vi "RT Loop - Watchdog.vi"(10 "FPGA VI Reference(Old)":T1, 11 "Message Queue":refnum<queue>) -> ()   [LabVIEW 2013]
uses:
  support/Message Queue/Message Cluster.ctl
  controls/FPGA VI Reference.ctl
  Globals/Global - Configuration Options.vi
  <vilib>/Utility/error.llb/Error Cluster From Error Code.vi
  <vilib>/rvi/errors/niLvFpgaAdjustHostInterfaceError.vi
  Globals/Global - All RT Loop Stop.vi
  <vilib>/rvi/interface/nirviReadWriteControl/nirviReadWriteControl.xnode
  FPGA Bitfiles/crio-FPGA-contro_FPGATarget_FPGAMain_4HKUk4gb9wY.lvbitx
  NiFpgaLv.dll
  support/Message Queue/Message Queue.lvlib
panel:
  in  "FPGA VI Reference":refnum<k20>
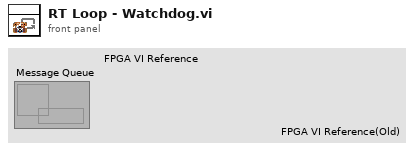
[diagram p1: front panel]
types:
  T1 = typedef "FPGA VI Reference.ctl" = refnum<k20>
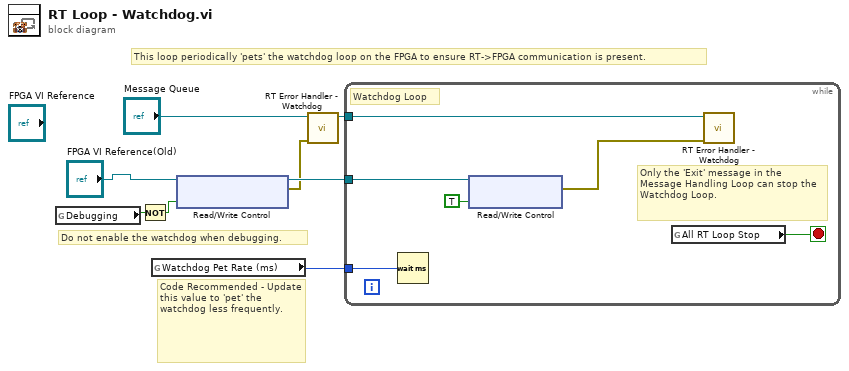
[diagram p0: block diagram]
diagram:
  # "Do not enable the watchdog when debugging."
  # "Code Recommended - Update this value to 'pet' the watchdog less frequently."
  # "This loop periodically 'pets' the watchdog loop on the FPGA to ensure RT->FPGA communication is present."
  n1 = global read "Global - Configuration Options.vi" "Debugging"() -> (w3:bool)
  n2 = Not(x=w3) -> (.not. x?=w2:bool)
  n3 = global read "Global - Configuration Options.vi" "Watchdog Pet Rate (ms)"() -> (w8:u32)
  n4 = xnode "Read/Write Control"("FPGA VI Reference In"="FPGA VI Reference(Old)", "Enable Watchdog"=w2) -> ("FPGA VI Reference Out"=w7:T1, "error out"=w4:errorcluster)  [unwired: 1 in]
  n5 = call "RT Error Handler - Watchdog.vi"("error in (no error)"=w4, "Message Queue"="Message Queue") -> ("dup Message Queue"=w5:refnum<queue>)  [unwired: 9 in]
  n6 = while {
    tunnel: w5 -> [w11]
    tunnel: w7 -> [w14]
    tunnel: w8 -> [w9]
    stop <- w12 stop-if-true
    # "Only the 'Exit' message in the  Message Handling Loop can stop the Watchdog Loop."
    # "Watchdog Loop"
    n7 = Wait (ms)(milliseconds to wait=w9) -> ()  [unwired: 1 out]
    n8 = xnode "Read/Write Control"("FPGA VI Reference In"=w14, "Pet Watchdog"=TRUE ("Pet RT Watchdog")) -> ("error out"=w10:errorcluster)  [unwired: 1 in, 1 out]
    n9 = global read "Global - All RT Loop Stop.vi" "All RT Loop Stop"() -> (w12:bool)
    n10 = call "RT Error Handler - Watchdog.vi"("error in (no error)"=w10, "Message Queue"=w11) -> ()  [unwired: 9 in, 1 out]
  }
